vi "Clear Window Position Cache.vi"(7 "Delete Empty File?":bool, 8 "error in (no error)":errorcluster, 10 "Path":path caption="Path (<User App Data>/<App Name>/Window Positions.ini)") -> (0 "error out":errorcluster)   [LabVIEW 2020, in "Panel.lvlib" / "Persistent Position.lvclass"]
doc: "Clears the current windows position cache.\n\n----\nPlease see the following web address for additional documentation and tutorial information:\nhttp://www.mooregoodideas.com/mgi-panel-manager/\n\nAuthor: Derek Trepanier\n\nCopyright (c) 2018, Moore Good Ideas, Inc.\n\nAll rights reserved.\n\nRedistribution and use in source and binary forms, with or without modification, are permitted provided that the following conditions are met:\n\n * Redistributions of source code must retain the above copyright notice, this list of conditions and the following disclaimer.\n * Redistributions in binary form must reproduce the above copyright notice, this list of conditions and the following disclaimer in the documentation and/or other materials provided with the distribution.\n * Neither the name of Moore Good Ideas, Inc. nor the names of its contributors may be used to endorse or promote products derived from this software without specific prior written permission.\n\nTHIS SOFTWARE IS PROVIDED BY THE COPYRIGHT HOLDERS AND CONTRIBUTORS \"AS IS\" AND ANY EXPRESS OR IMPLIED WARRANTIES, INCLUDING, BUT NOT LIMITED TO, THE IMPLIED WARRANTIES OF MERCHANTABILITY AND FITNESS FOR A PARTICULAR PURPOSE ARE DISCLAIMED. IN NO EVENT SHALL THE COPYRIGHT OWNER OR CONTRIBUTORS BE LIABLE FOR ANY DIRECT, INDIRECT, INCIDENTAL, SPECIAL, EXEMPLARY, OR CONSEQUENTIAL DAMAGES (INCLUDING, BUT NOT LIMITED TO, PROCUREMENT OF SUBSTITUTE GOODS OR SERVICES; LOSS OF USE, DATA, OR PROFITS; OR BUSINESS INTERRUPTION) HOWEVER CAUSED AND ON ANY THEORY OF LIABILITY, WHETHER IN CONTRACT, STRICT LIABILITY, OR TORT (INCLUDING NEGLIGENCE OR OTHERWISE) ARISING IN ANY WAY OUT OF THE USE OF THIS SOFTWARE, EVEN IF ADVISED OF THE POSSIBILITY OF SUCH DAMAGE."
uses:
  <vilib>/MGI/Panel Manager/Panel/Window Position/Persistent Position/Persistent Position.lvclass
  <vilib>/Utility/config.llb/NI_LVConfig.lvlib
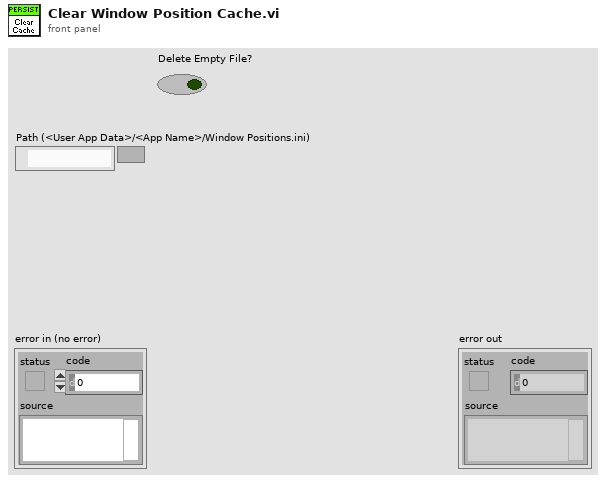
[diagram p1: front panel]
types:
  T1 = typedef "NI_LVConfig.lvlib/Config Data RefNum.ctl" = refnum<k1>
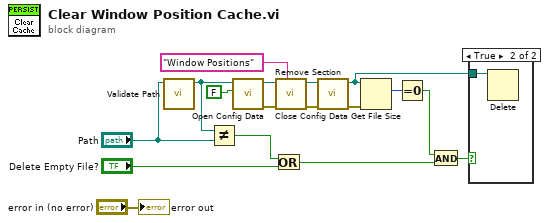
[diagram p0: block diagram]
diagram:
  n1 = call <vilib>:"Validate Path.vi"("Path in"="Path") -> ("Path out"=w9:path)  [unwired: 10 in]
  n2 = Not Equal?(x=w9, y="Path") -> (x != y?=w7:bool)
  n3 = call <vilib>:"Open Config Data.vi"("create file if necessary (T)"=FALSE, "configuration file path"=w9) -> ("error out"=w12:errorcluster, "refnum"=w15:T1)  [unwired: 7 in, 1 out]
  n4 = Or(x=w7, y="Delete Empty File?") -> (x .or. y?=w3:bool)
  n5 = call <vilib>:"Remove Section.vi"("section"="Window Positions", "error in (no error)"=w12, "refnum"=w15) -> ("error out"=w13:errorcluster, "refnum out"=w14:T1)  [unwired: 6 in, 1 out]
  n6 = call <vilib>:"Close Config Data.vi"("error in (no error)"=w13, "refnum"=w14) -> ("error out"=w10:errorcluster, "file path"=w1:path)  [unwired: 8 in]
  n7 = Get File Size(file=w1, error in=w10) -> (size (in bytes)=w5:i64)  [unwired: 2 out]
  n8 = Equal To 0?(x=w5) -> (x = 0?=w4:bool)
  n9 = And(x=w4, y=w3) -> (x .and. y?=w2:bool)
  n10 = case shown="True" w2 {
    tunnel: w1 -> [_ w18]
    frame False {
    }
    frame True {
      n11 = Delete(path (use dialog)=w18) -> ()  [unwired: 4 in, 3 out]
    }
  }
  "error out" <- "error in (no error)"
